vi "readTCPDataIn.vi"(8 "error in (no error)":errorcluster, 10 "Size of data":string, 11 "TCP Network Connection in":refnum<k5>) -> (0 "error out":errorcluster, 1 "Data":string, 2 "Operation":string, 3 "TCP Network Connection out":refnum<k5>)   [LabVIEW 2015]
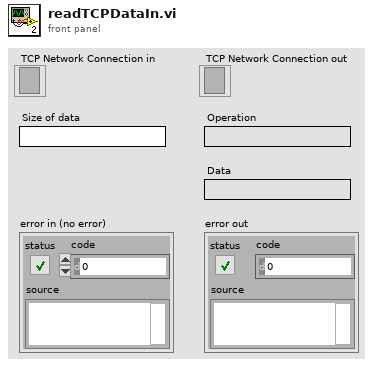
[diagram p1: front panel]
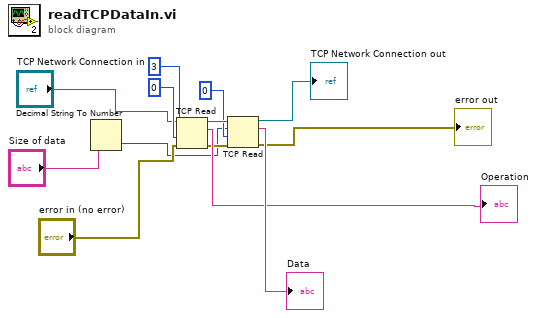
[diagram p0: block diagram]
diagram:
  n1 = Decimal String To Number(string="Size of data") -> (number=w5:i32)  [unwired: 2 in, 1 out]
  n2 = TCP Read(connection ID="TCP Network Connection in", bytes to read=3, error in (no error)="error in (no error)", 9:0 ("timeout ms (25000)")) -> (connection ID out=w7:refnum<k5>, data out=→"Operation":string, error out=w9:errorcluster)  [unwired: 1 in]
  n3 = TCP Read(connection ID=w7, bytes to read=w5, error in (no error)=w9, 9:0 ("timeout ms (25000)")) -> (connection ID out=→"TCP Network Connection out":refnum<k5>, data out=→"Data":string, error out=→"error out":errorcluster)  [unwired: 1 in]
